vi "Stop.vi"(8 "error in (no error)":errorcluster, 11 "AODAcq in":refnum<class "AODAcq.lvclass">) -> (0 "error out":errorcluster, 3 "AODAcq out":refnum<class "AODAcq.lvclass">)   [LabVIEW 2011, in "AODAcq.lvclass"]
uses:
  AODAcq.lvclass
  <vilib>/Utility/error.llb/Error Cluster From Error Code.vi
  <vilib>/rvi/errors/niLvFpgaAdjustHostInterfaceError.vi
  <vilib>/rvi/interface/nirviMethod/nirviMethod.xnode
  FPGA_Control/AODRef.ctl
  FPGA Bitfiles/Acquisition_FPGATarget_AODControl(FPGA)_C1C38267.lvbitx
  FPGA_Control/AOD Control (FPGA).vi
  HDF5Tools/LabView/HDF5Tools.lvlib
  <vilib>/FPGAPlugInAG/PXIe-7965R/niLvFpga_ReadFifo_PXIe-7965R.vi
  <vilib>/rvi/errors/niLvFpgaMergeErrorWithErrorCode.vi
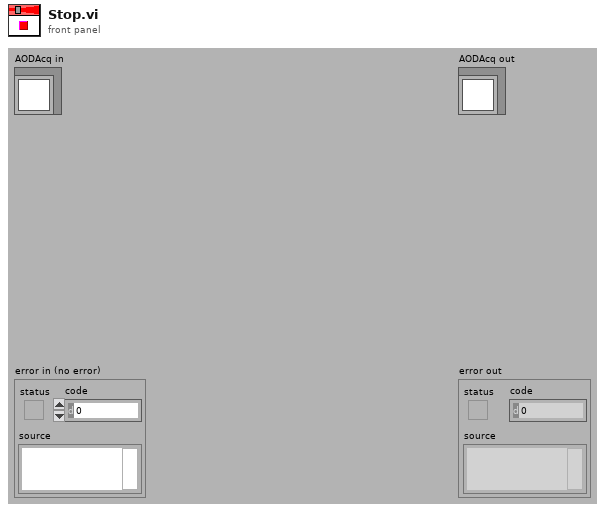
[diagram p1: front panel]
types:
  T1 = cluster{"file handle out":i32, "ImData":i32, "TemporalData":i32, "MotionData":i32}
  T2 = typedef "AODRef.ctl" = refnum<k20>
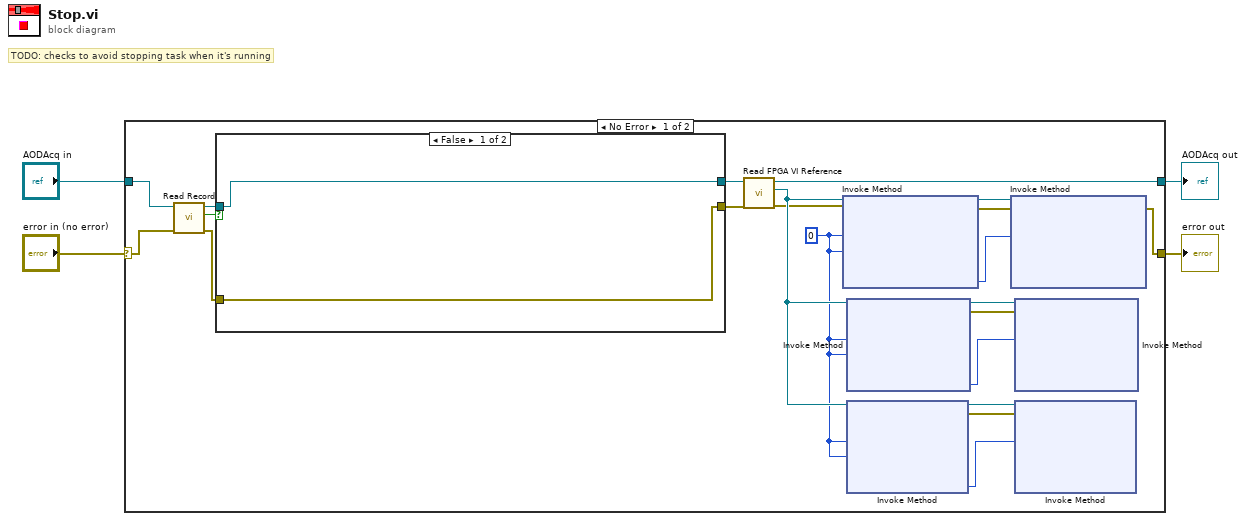
[diagram p0: block diagram]
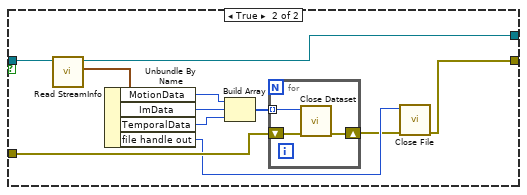
[diagram p2: hidden frame]
diagram:
  # "TODO: checks to avoid stopping task when it's running"
  n1 = case shown="No Error" "error in (no error)" {
    selector: "error in (no error)" -> [w10 w43]
    tunnel: [w12 w43] -> w3
    tunnel: [w14 w42] -> w1
    tunnel: "AODAcq in" -> [w9 w42]
    frame No Error {
      w18 = u32 0 ("Number of Elements")
      n2 = call-dynamic "Read Record.vi"("error in (no error)"=w10, "AODAcq in"=w9) -> ("error out"=w6:errorcluster, "Record"=w7:bool, "AODAcq out"=w8:refnum<class "AODAcq.lvclass">)  [unwired: 7 in]
      n3 = case shown="False" w7 {
        tunnel: [w26 w38] -> w11
        tunnel: w8 -> [w26 w37]
        tunnel: w6 -> [w27 w31]
        tunnel: [w27 w28] -> w5
        frame False {
        }
        frame True {
          n4 = call-dynamic "Read StreamInfo.vi"("AODAcq in"=w37) -> ("StreamInfo"=w36:T1, "AODAcq out"=w38:refnum<class "AODAcq.lvclass">)  [unwired: 8 in, 1 out]
          n5 = Unbundle By Name(w36) -> ("MotionData"=w33:i32, "ImData"=w34:i32, "TemporalData"=w35:i32, "file handle out"=w30:i32)
          n6 = Build Array(w33, w34, w35) -> (w32:i32[])
          n7 = for {
            tunnel: w32 -> [w41] mode=indexing
            shift-right: [w39] -> w29
            shift-left: w31 -> [w40]
            n8 = call "Close Dataset.vi"("error in (no error)"=w40, "dataset_id"=w41) -> ("error out"=w39:errorcluster)  [unwired: 9 in]
          }
          n9 = call "Close File.vi"("error in (no error)"=w29, "file_id"=w30) -> ("error out"=w28:errorcluster)  [unwired: 9 in]
        }
      }
      n10 = call-dynamic "Read FPGA VI Reference.vi"("error in (no error)"=w5, "AODAcq in"=w11) -> ("error out"=w13:errorcluster, "FPGA VI Reference"=w25:T2, "AODAcq out"=w14:refnum<class "AODAcq.lvclass">)  [unwired: 7 in]
      n11 = xnode "Invoke Method"("FPGA VI Reference In"=w25, "error in"=w13, "Number of Elements"=w18, "Timeout (ms)"=w18) -> ("FPGA VI Reference Out"=w24:T2, "error out"=w23:errorcluster, "Elements Remaining"=w15:u32)  [unwired: 1 out]
      n12 = xnode "Invoke Method"("FPGA VI Reference In"=w25, "Number of Elements"=w18, "Timeout (ms)"=w18) -> ("FPGA VI Reference Out"=w22:T2, "error out"=w21:errorcluster, "Elements Remaining"=w16:u32)  [unwired: 1 in, 1 out]
      n13 = xnode "Invoke Method"("FPGA VI Reference In"=w25, "Number of Elements"=w18, "Timeout (ms)"=w18) -> ("FPGA VI Reference Out"=w20:T2, "error out"=w19:errorcluster, "Elements Remaining"=w17:u32)  [unwired: 1 in, 1 out]
      n14 = xnode "Invoke Method"("FPGA VI Reference In"=w24, "error in"=w23, "Number of Elements"=w15) -> ("error out"=w12:errorcluster)  [unwired: 1 in, 3 out]
      n15 = xnode "Invoke Method"("FPGA VI Reference In"=w22, "error in"=w21, "Number of Elements"=w16) -> ()  [unwired: 1 in, 4 out]
      n16 = xnode "Invoke Method"("FPGA VI Reference In"=w20, "error in"=w19, "Number of Elements"=w17) -> ()  [unwired: 1 in, 4 out]
    }
    frame Error {
    }
  }
  "error out" <- w3
  "AODAcq out" <- w1
